vi "PH_PP_CurrentMeas.PC set Data to GUI.vi"(2 "Ref GUI element":refnum<vi>, 3 "Data":waveform(dbl)[](array[waveform]), 4 "error in (no error)":errorcluster) -> (18 "error out":errorcluster)   [LabVIEW 2014, in "PH_PP_CurrentMeas.lvlib"]
doc: "This VI indicates the data at the GUI. It scales the data with a factor of 0.66 in order to indicate the data in kA."
uses:
  PH_PP_CurrentMeas.lvlib
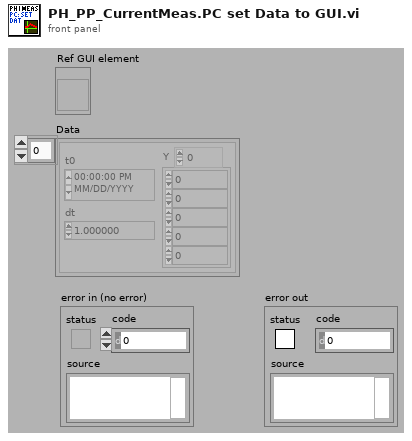
[diagram p1: front panel]
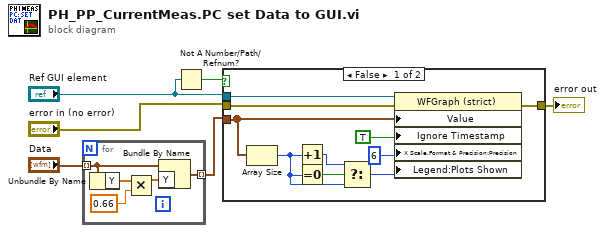
[diagram p0: block diagram]
diagram:
  n1 = for {
    tunnel: "Data" -> [w7] mode=indexing
    tunnel: [w8] -> w1 mode=indexing
    n2 = Unbundle By Name(w7) -> ("Y"=w11:dbl[])
    n3 = Multiply(x=w11, y=0.66) -> (x*y=w9:dbl[])
    n4 = Bundle By Name(cluster=w7, "Y"=w9) -> (w8:waveform(dbl))
  }
  n5 = Not A Number/Path/Refnum?(number/path/refnum="Ref GUI element") -> (NaN/Path/Refnum?=w4:bool)
  n6 = case shown="False" w4 {
    tunnel: "Ref GUI element" -> [w21 _]
    tunnel: w1 -> [w16 _]
    tunnel: "error in (no error)" -> [w20 w22]
    tunnel: [w19 w22] -> w3
    frame False {
      n7 = Array Size(array=w16) -> (size(s)=w13:i32)
      n8 = Increment(x=w13) -> (x+1=w14:i32)
      n9 = Equal To 0?(x=w13) -> (x = 0?=w15:bool)
      n10 = Select(t=w14, s=w15, f=w13) -> (s? t:f=w12:i32)
      n11 = property class="WFGraph (strict)"(reference=w21, error in=w20, "Value"=w16, "Ignore Timestamp"=TRUE, "X Scale.Format & Precision:Precision"=u8 6, "Legend:Plots Shown"=w12) -> (error out=w19:errorcluster)  [unwired: 1 out]
    }
    frame True {
    }
  }
  "error out" <- w3
